vi "Initialize.vi"(7 "Channel Name":string="ActualValue.ch%d.AV", 8 "error in":errorcluster, 9 "Number of Channels":u32=1, 10 "Instance Name":string, 11 "Humidity Actual Value in":refnum<class "Humidity Actual Value.lvclass">) -> (0 "error out":errorcluster, 3 "Humidity Actual Value out":refnum<class "Humidity Actual Value.lvclass">)   [LabVIEW 2023, in "Humidity Actual Value.lvclass"]
uses:
  Humidity Actual Value.lvclass
  Parents/Actual Value/Actual Value.lvclass
  Humidity Actual Value.lvclass/Humidity Actual Value.ctl
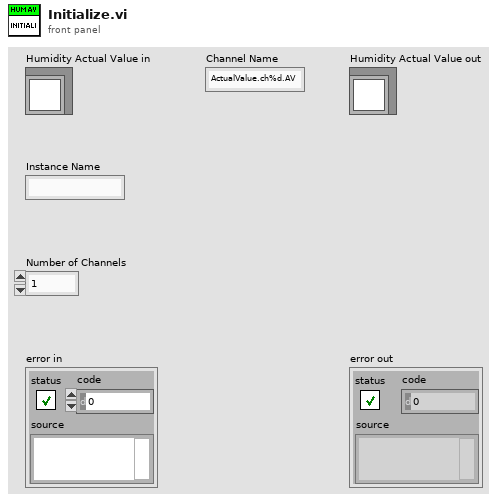
[diagram p1: front panel]
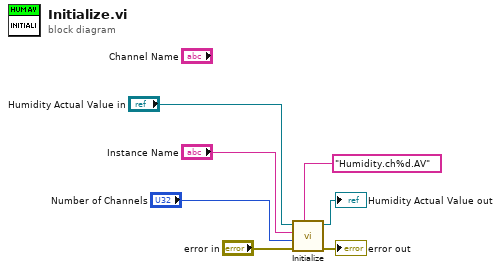
[diagram p0: block diagram]
diagram:
  n1 = call-parent "Initialize.vi"("Channel Name"="Humidity.ch%d.AV", "error in"="error in", "Number of Channels"="Number of Channels", "Instance Name"="Instance Name", "Actual Value in"="Humidity Actual Value in") -> ("error out"=→"error out":errorcluster, "Actual Value out"=→"Humidity Actual Value out":refnum<class "Humidity Actual Value.lvclass">)  [unwired: 5 in]
